vi "ExitationIntensityTrace.vi"(5 "error in 2":errorcluster) -> (17 "data":dbl format="%.2f", 19 "error out":errorcluster)   [LabVIEW 2011]
uses:
  <vilib>/DAQmx/read.llb/DAQmx Read (Analog DBL 1Chan 1Samp).vi
  <vilib>/DAQmx/create/channels.llb/DAQmx Create Channel (AI-Voltage-Basic).vi
  <vilib>/DAQmx/miscellaneous.llb/DAQmx Fill In Error Info.vi
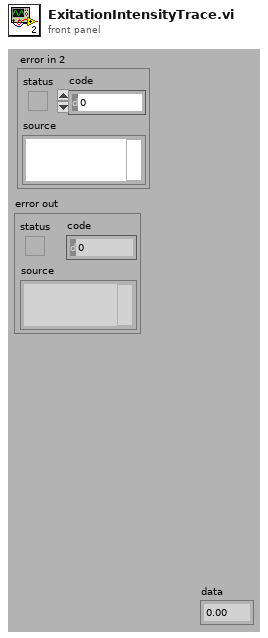
[diagram p1: front panel]
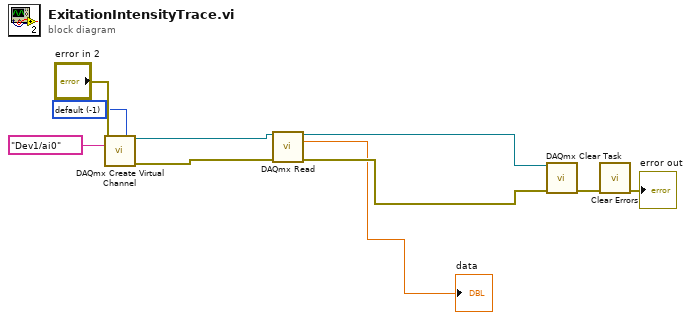
[diagram p0: block diagram]
diagram:
  w2 = -1 items=["default"=-1, "RSE"=10083, "NRSE"=10078, "Differential"=10106, "Pseudodifferential"=12529] ("input terminal configuration")
  n1 = call-poly <vilib>:"DAQmx Create Virtual Channel.vi"("input terminal configuration"=w2, "physical channels"=tag "Dev1/ai0", "error in"="error in 2") -> ("task out"=w4:refnum<k21>, "error out"=w5:errorcluster)  [unwired: 11 in]
  n2 = call-poly <vilib>:"DAQmx Read.vi"("task/channels in"=w4, "error in"=w5) -> ("task out"=w8:refnum<k21>, "data"=→"data":dbl, "error out"=w7:errorcluster)  [unwired: 11 in]
  n3 = call <vilib>:"DAQmx Clear Task.vi"("task in"=w8, "error in"=w7) -> ("error out"=w6:errorcluster)  [unwired: 13 in]
  n4 = call <vilib>:"Clear Errors.vi"("error in (no error)"=w6) -> ("error out"=→"error out":errorcluster)  [unwired: 6 in]
